vi "LWXPS_DebugTraceCommunicationReset.vi"(6 "LabVIEW error IN":errorcluster, 9 "XPS Reference IN":refnum<k24>) -> (0 "LabVIEW error OUT":errorcluster, 1 "XPS Error String":string, 2 "Returned error code":i32, 3 "XPS Reference OUT":refnum<k24>)   [LabVIEW 2014]
uses:
  D:/XPSQ8_LabView_Library/Development/Source/Dll/Newport.XPS.CommandInterface.dll
  Dll/Newport.XPS.CommandInterface.dll
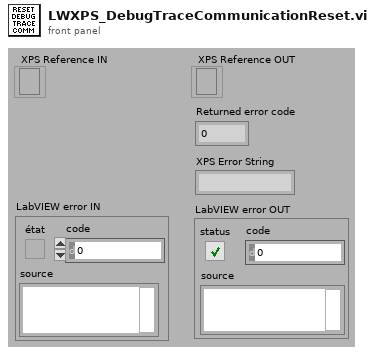
[diagram p1: front panel]
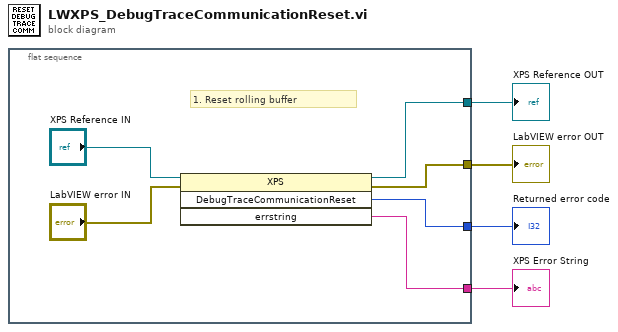
[diagram p0: block diagram]
diagram:
  n1 = flat-sequence {
    tunnel: [w7] -> w4
    tunnel: [w10] -> w3
    tunnel: [w6] -> w2
    tunnel: [w5] -> w1
    frame #0 {
      # "1. Reset rolling buffer"
      n2 = invoke class="XPS" method="DebugTraceCommunicationReset"(reference="XPS Reference IN", error in="LabVIEW error IN") -> (reference out=w7:refnum<k24>, error out=w10:errorcluster, "DebugTraceCommunicationReset"=w6:i32, "errstring"=w5:string)  [unwired: 2 in]
    }
  }
  "XPS Reference OUT" <- w4
  "LabVIEW error OUT" <- w3
  "Returned error code" <- w2
  "XPS Error String" <- w1
